vi "Build Target Sections.vi"(6 "Add Legal Section":bool, 8 "error in":errorcluster, 10 "Target":T1) -> (0 "error out":errorcluster, 3 "Target Sections":refnum<class "Section.lvclass">[](array[class]))   [LabVIEW 2021, in "TAF Proj Document Type.lvlib" / "TAF Proj.lvclass"]
uses:
  <vilib>/Wovalab/AntiDoc/Document Type/Add-ons/LabVIEW TAF Project/TAF Proj/TAF Proj.lvclass
  <vilib>/Wovalab/AntiDoc/Section/Section.lvclass
  <vilib>/Wovalab/AntiDoc/Document Type/Add-ons/LabVIEW TAF Project/Project Parser/Target--cluster.ctl
  <vilib>/Wovalab/AntiDoc/Document Type/Add-ons/LabVIEW TAF Project/Custom Errors/Custom Errors.lvclass
  <vilib>/Wovalab/AntiDoc/Document Type/Add-ons/LabVIEW TAF Project/Classes Overview/Classes Overview.lvclass
  <vilib>/Wovalab/AntiDoc/Document Type/Add-ons/LabVIEW TAF Project/Dqmh Modules Overview/Dqmh Modules Overview.lvclass
  <vilib>/Wovalab/AntiDoc/Document Type/Add-ons/LabVIEW TAF Project/FrontPanelGUI/FrontPanelGUI.lvclass
  <vilib>/Wovalab/AntiDoc/Document Type/Add-ons/LabVIEW TAF Project/Project Parser/Blocs--cluster.ctl
  <vilib>/Wovalab/AntiDoc/Document Type/Add-ons/LabVIEW TAF Project/Dqmh Module/Dqmh Module.lvclass
  <vilib>/Wovalab/AntiDoc/Document Type/Add-ons/LabVIEW TAF Project/Class/Class.lvclass
  C:/Program Files (x86)/National Instruments/LabVIEW 2021/vi.lib/Wovalab/AntiDoc/Document Type/Add-ons/LabVIEW YAF Project/Lib/Lib.lvclass
  <vilib>/Wovalab/AntiDoc/Document Type/Add-ons/LabVIEW TAF Project/Lib/Lib.lvclass
  <vilib>/Wovalab/AntiDoc/Document Type/Add-ons/LabVIEW TAF Project/TAFConfiguration/TAFConfiguration.lvclass
  <vilib>/Wovalab/AntiDoc/Sub Section/Sub Section.lvclass
  C:/Program Files (x86)/National Instruments/LabVIEW 2021/vi.lib/Wovalab/AntiDoc/Section/Section.lvclass
  <vilib>/Wovalab/AntiDoc/Document Type/Add-ons/LabVIEW TAF Project/Project Parser/Project Parser.lvlib
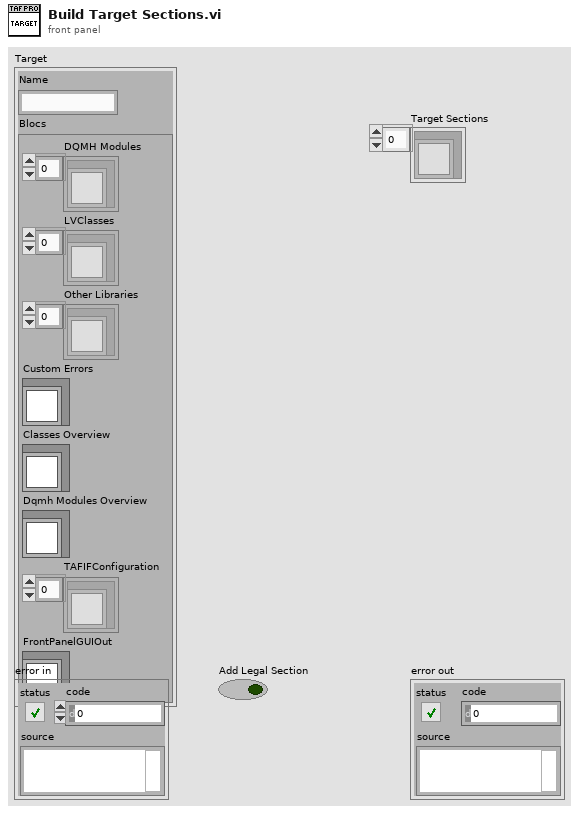
[diagram p1: front panel]
types:
  T1 = typedef "TAF Proj Document Type.lvlib/Project Parser.lvlib/Target--cluster.ctl" = cluster{"Name":string, "Blocs":T2}
  T2 = typedef "TAF Proj Document Type.lvlib/Project Parser.lvlib/Blocs--cluster.ctl" = cluster{"DQMH Modules":refnum<class "Dqmh Module.lvclass">[], "LVClasses":refnum<class "Class.lvclass">[], "Other Libraries":refnum<class "Lib.lvclass">[], "Custom Errors":refnum<class "Custom Errors.lvclass">, "Classes Overview":refnum<class "Classes Overview.lvclass">, "Dqmh Modules Overview":refnum<class "Dqmh Modules Overview.lvclass">, "TAFIFConfiguration":refnum<class "TAFConfiguration.lvclass">[], "FrontPanelGUIOut":refnum<class "FrontPanelGUI.lvclass">}
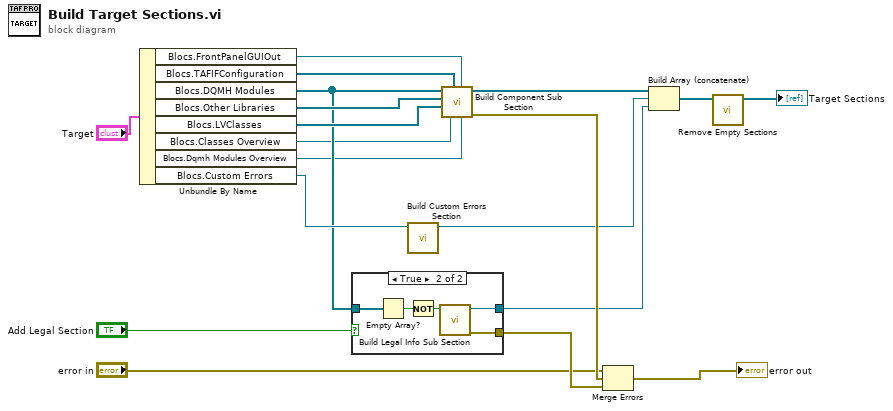
[diagram p0: block diagram]
diagram:
  n1 = Unbundle By Name("Target") -> ("Blocs.FrontPanelGUIOut"=w1:refnum<class "FrontPanelGUI.lvclass">, "Blocs.TAFIFConfiguration"=w2:refnum<class "TAFConfiguration.lvclass">[], "Blocs.DQMH Modules"=w10:refnum<class "Dqmh Module.lvclass">[], "Blocs.Other Libraries"=w11:refnum<class "Lib.lvclass">[], "Blocs.LVClasses"=w12:refnum<class "Class.lvclass">[], "Blocs.Classes Overview"=w6:refnum<class "Classes Overview.lvclass">, "Blocs.Dqmh Modules Overview"=w3:refnum<class "Dqmh Modules Overview.lvclass">, "Blocs.Custom Errors"=w13:refnum<class "Custom Errors.lvclass">)
  n2 = case shown="True" "Add Legal Section" {
    tunnel: [_ w24] -> w19
    tunnel: w10 -> [_ w23]
    tunnel: [_ w20] -> w9
    frame False {
    }
    frame True {
      n3 = Empty Array?(array=w23) -> (empty?=w21:bool)
      n4 = Not(x=w21) -> (.not. x?=w22:bool)
      n5 = call <vilib>:"Build Legal Info Sub Section.vi"("Has DQMH modules"=w22) -> ("error out"=w24:errorcluster, "Lv Proj Document Type:TAF Proj"=w20:refnum<class "Sub Section.lvclass">)  [unwired: 9 in]
    }
  }
  n6 = call <vilib>:"Build Custom Errors Section.vi"("Lv Proj Document Type:TAF Proj"=w13) -> ("Lv Proj Document Type:TAF Proj"=w14:refnum<class "Section.lvclass">)  [unwired: 9 in, 1 out]
  n7 = call <vilib>:"Build Component Sub Section.vi"("Dqmh Modules Overview"=w3, "FrontPanelGUIOut"=w1, "Classes Overview"=w6, "TAFConfiguration"=w2, "Lvclass"=w12, "Libraries"=w11, "Dqmh Modules"=w10) -> ("error out"=w18:errorcluster, "Sections"=w8:refnum<class "Section.lvclass">[])  [unwired: 3 in]
  n8 = Merge Errors("error in", w18, w19) -> (→"error out":errorcluster)
  n9 = Build Array (concatenate)(w8, w14, w9) -> (w5:refnum<class "Section.lvclass">[])
  n10 = call <vilib>:"Remove Empty Sections .vi"("Array in"=w5) -> ("Array out"=→"Target Sections":refnum<class "Section.lvclass">[])  [unwired: 10 in]
